vi "Words To Network-Order Bytes Poly.vi"   [LabVIEW 2020, in "NI_Bit Manipulation.lvlib"]
doc: "Convert an integer to a byte array in network byte order, i.e., big-endian. This polymorphic VI wraps an underlying malleable VI."
uses:
  <vilib>/Bit Manipulation/NI_Bit Manipulation.lvlib
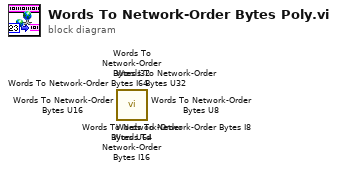
[diagram p0: block diagram]
diagram:
  n1 = call <vilib>:"Words To Network-Order Bytes U64.vi"() -> ()  [unwired: 1 in, 1 out]
  n2 = call <vilib>:"Words To Network-Order Bytes U32.vi"() -> ()  [unwired: 1 in, 1 out]
  n3 = call <vilib>:"Words To Network-Order Bytes U16.vi"() -> ()  [unwired: 1 in, 1 out]
  n4 = call <vilib>:"Words To Network-Order Bytes U8.vi"() -> ()  [unwired: 1 in, 1 out]
  n5 = call <vilib>:"Words To Network-Order Bytes I64.vi"() -> ()  [unwired: 1 in, 1 out]
  n6 = call <vilib>:"Words To Network-Order Bytes I32.vi"() -> ()  [unwired: 1 in, 1 out]
  n7 = call <vilib>:"Words To Network-Order Bytes I16.vi"() -> ()  [unwired: 1 in, 1 out]
  n8 = call <vilib>:"Words To Network-Order Bytes I8.vi"() -> ()  [unwired: 1 in, 1 out]
